vi "valve_control.vi"(5 "Set new position":bool, 10 "Valve set pos (deg, 0-90)":i8, 11 "VISA resource name":refnum<visa-resource-name>="COM1") -> (2 "Valve position (deg, 0-90)):":string)   [LabVIEW 2018]
uses:
  <vilib>/Instr/_visa.llb/VISA Configure Serial Port (Instr).vi
panel:
  out "Valve ID:":string
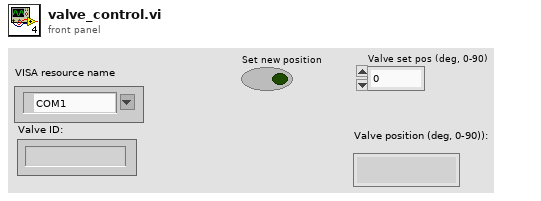
[diagram p1: front panel]
types:
  T1 = cluster{"baud rate":u32, "data bits":u16, "parity":enum16{"None", "Odd", "Even", "Mark", "Space"}, "stop bits":u16, "flow control":u16}
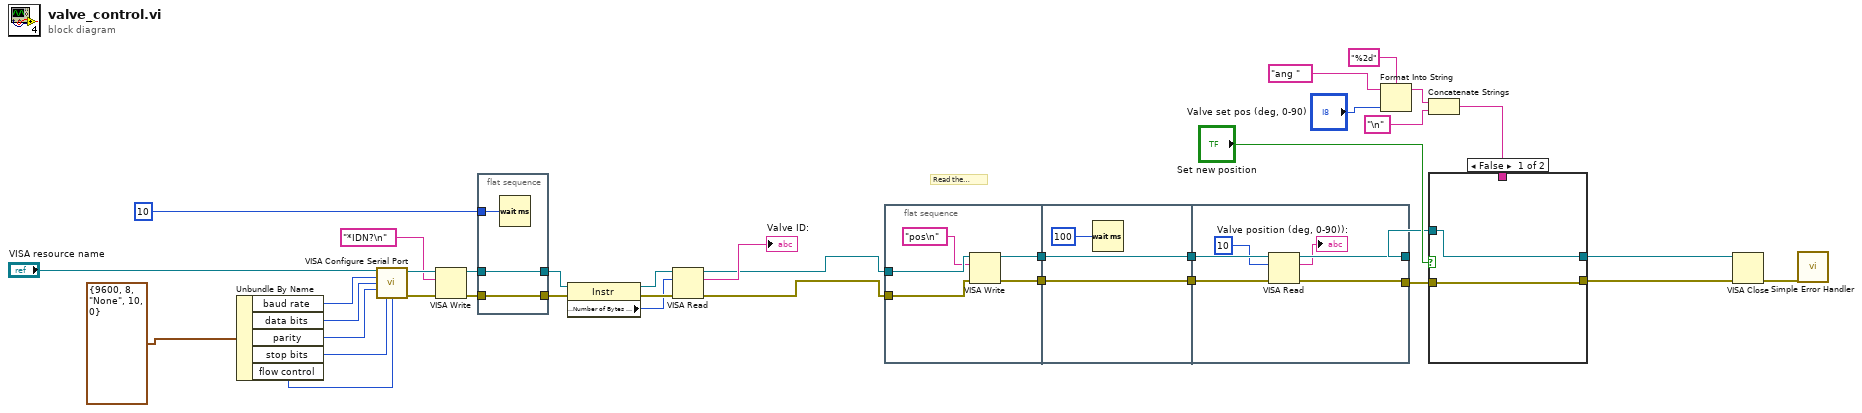
[diagram p0: block diagram]
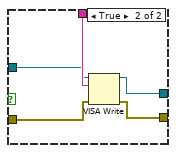
[diagram p2: hidden frame]
diagram:
  # "Read the position"
  n1 = Unbundle By Name(T1 {"baud rate"=9600, "data bits"=8, "parity"=enum."None", "stop bits"=10, "flow control"=0} ("Serial Settings")) -> ("baud rate"=w23:u32, "data bits"=w22:u16, "parity"=w21:enum16{"None", "Odd", "Even", "Mark", "Space"}, "stop bits"=w20:u16, "flow control"=w19:u16)
  n2 = call-poly "VISA Configure Serial Port"("VISA resource name"="VISA resource name", "baud rate (9600)"=w23, "data bits (8)"=w22, "parity (0:none)"=w21, "stop bits (10: 1 bit)"=w20, "flow control (0:none)"=w19) -> ("VISA resource name out"=w35:refnum<visa-resource-name>, "error out"=w36:errorcluster)  [unwired: 3 in, 5 out]
  n3 = VISA Write(VISA resource name=w35, write buffer="*IDN?\n" ("Command"), error in (no error)=w36) -> (VISA resource name out=w31:refnum<visa-resource-name>, error out=w33:errorcluster)  [unwired: 1 out]
  n4 = flat-sequence {
    tunnel: w33 -> [w39]
    tunnel: [w39] -> w32
    tunnel: w31 -> [w38]
    tunnel: [w38] -> w30
    tunnel: u32 10 ("delay before read (ms)") -> [w40]
    frame #0 {
      n5 = Wait (ms)(milliseconds to wait=w40) -> ()  [unwired: 1 out]
    }
  }
  n6 = property class="Instr"(reference=w30, error in=w32) -> (reference out=w27:refnum<visa-resource-name>, error out=w26:errorcluster, "Serial Settings:Number of Bytes at Serial Port"=w24:u32)
  n7 = VISA Read(VISA resource name=w27, byte count=w24, error in (no error)=w26) -> (VISA resource name out=w18:refnum<visa-resource-name>, read buffer=→"Valve ID:":string, error out=w17:errorcluster)  [unwired: 1 out]
  n8 = flat-sequence {
    tunnel: w18 -> [w45]
    tunnel: w17 -> [w44]
    tunnel: [w43] -> w13
    tunnel: [w42] -> w12
    tunnel: w13 -> [w48]
    tunnel: [w48] -> w11
    tunnel: w12 -> [w47]
    tunnel: [w47] -> w10
    tunnel: [w50] -> w1
    tunnel: w11 -> [w54]
    tunnel: w10 -> [w53]
    tunnel: [w51] -> w2
    frame #0 {
      n9 = VISA Write(VISA resource name=w45, write buffer="pos\n" ("Command"), error in (no error)=w44) -> (VISA resource name out=w42:refnum<visa-resource-name>, error out=w43:errorcluster)  [unwired: 1 out]
    }
    frame #1 {
      n10 = Wait (ms)(milliseconds to wait=u32 100) -> ()  [unwired: 1 out]
    }
    frame #2 {
      n11 = VISA Read(VISA resource name=w53, byte count=u32 10, error in (no error)=w54) -> (VISA resource name out=w51:refnum<visa-resource-name>, read buffer=→"Valve position (deg, 0-90)):":string, error out=w50:errorcluster)  [unwired: 1 out]
    }
  }
  n12 = Format Into String(format string="%2d", initial string="ang " ("Command"), "Valve set pos (deg, 0-90)") -> (resulting string=w4:string)  [unwired: 1 in, 1 out]
  n13 = Concatenate Strings(w4, "\n" ("Command")) -> (w3:string)
  n14 = case shown="False" "Set new position" {
    tunnel: w3 -> [_ w61]
    tunnel: w2 -> [w56 w60]
    tunnel: w1 -> [w55 w59]
    tunnel: [w56 w58] -> w16
    tunnel: [w55 w57] -> w15
    frame False {
    }
    frame True {
      n15 = VISA Write(VISA resource name=w60, write buffer=w61, error in (no error)=w59) -> (VISA resource name out=w58:refnum<visa-resource-name>, error out=w57:errorcluster)  [unwired: 1 out]
    }
  }
  n16 = VISA Close(VISA resource name=w16, error in (no error)=w15) -> (error out=w34:errorcluster)
  n17 = call <vilib>:"Simple Error Handler.vi"("error in (no error)"=w34) -> ()  [unwired: 1 in, 8 out]
